vi "SELECT Income and Expenses.vi"(8 "error in (no error)":errorcluster, 9 "Month":T1, 10 "YYYY":i32, 11 "Database in":refnum<class "Database.lvclass">) -> (0 "error out":errorcluster, 1 "Total Expenses":dbl, 2 "Total Income":dbl, 3 "Database out":refnum<class "Database.lvclass">)   [LabVIEW 2018, in "Database.lvclass"]
uses:
  Database.lvclass
  Month.ctl
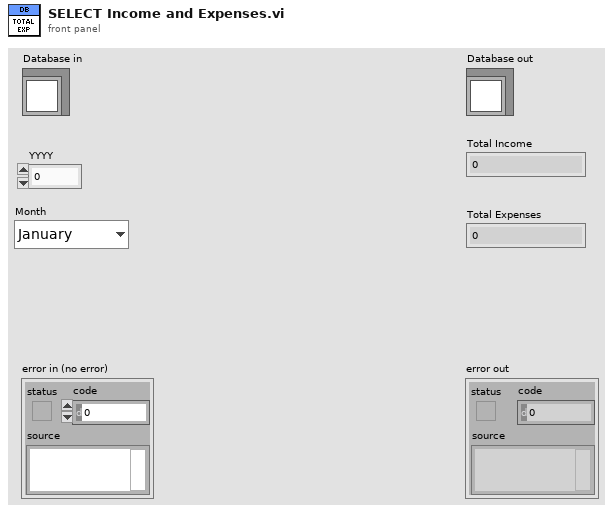
[diagram p1: front panel]
types:
  T1 = typedef "Database.lvclass/Month.ctl" = enum16{"January", "February", "March", "April", "May", "June", "July", "August", "September", "October", "November", "December"}
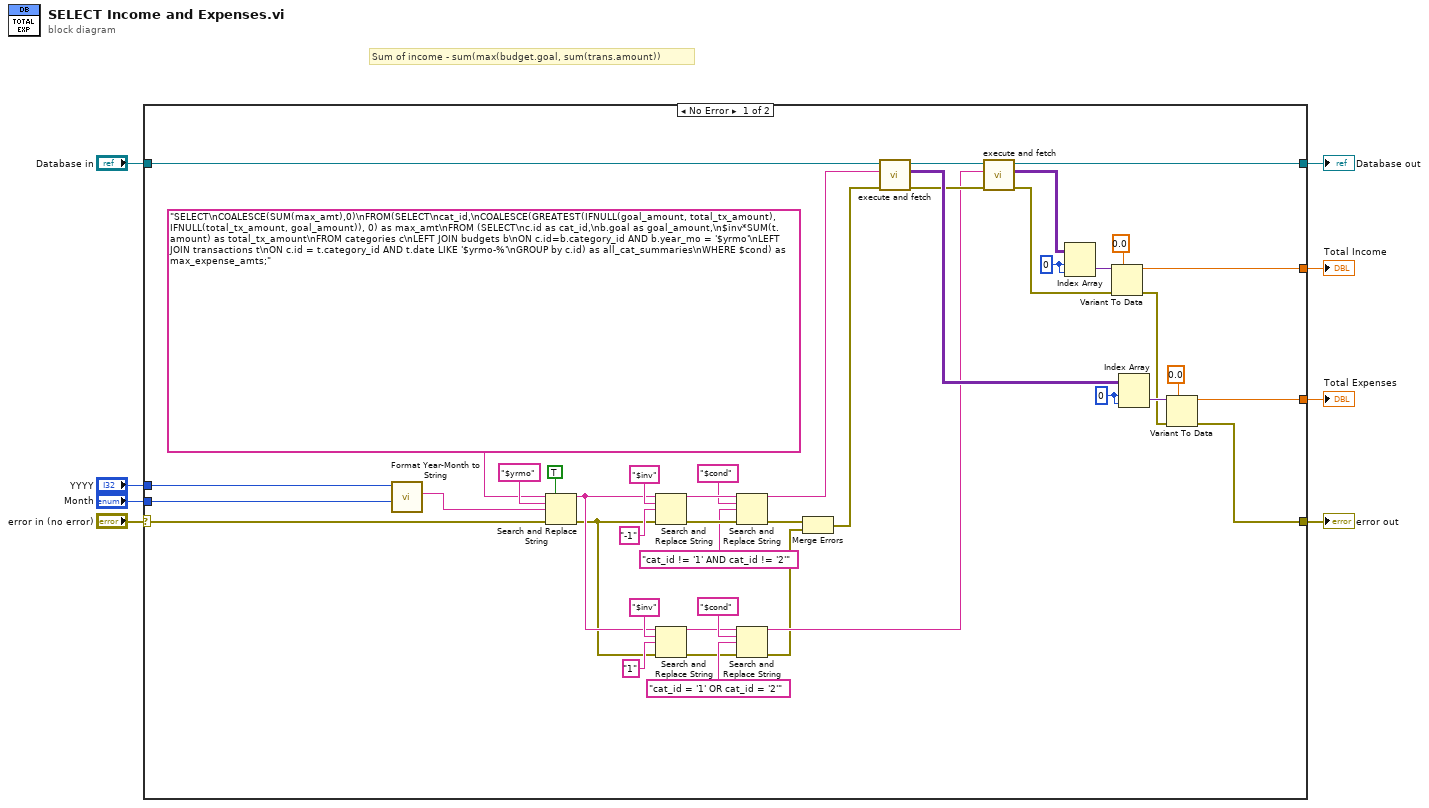
[diagram p0: block diagram]
diagram:
  # "Sum of income - sum(max(budget.goal, sum(trans.amount))"
  n1 = case shown="No Error" "error in (no error)" {
    selector: "error in (no error)" -> [w25 w53]
    tunnel: [w41 w53] -> w7
    tunnel: [w14 w52] -> w5
    tunnel: "Database in" -> [w51 w52]
    tunnel: "YYYY" -> [w50 _]
    tunnel: "Month" -> [w49 _]
    tunnel: [w40 _] -> w2
    tunnel: [w15 _] -> w1
    frame No Error {
      w17 = 0 ("index (row)")
      w44 = 0 ("index (row)")
      n2 = call "Format Year-Month to String.vi"("Month"=w49, "YYYY"=w50) -> ("Year-Mo"=w46:string)  [unwired: 9 in]
      n3 = Search and Replace String(replace all?=TRUE ("replace all? (F)"), input string="SELECT\nCOALESCE(SUM(max_amt),0)\nFROM(SELECT\ncat_id,\nCOALESCE(GREATEST(IFNULL(goal_amount, total_tx_amount), IFNULL(total_tx_amount, goal_amount)), 0) as max_amt\nFROM (SELECT\nc.id as cat_id,\nb.goal as goal_amount,\n$inv*SUM(t.amount) as total_tx_amount\nFROM categories c\nLEFT JOIN budgets b\nON c.id=b.category_id AND b.year_mo = '$yrmo'\nLEFT JOIN transactions t\nON c.id = t.category_id AND t.date LIKE '$yrmo-%'\nGROUP by c.id) as all_cat_summaries\nWHERE $cond) as max_expense_amts;", search string="$yrmo", replace string=w46, error in=w25) -> (result string=w24:string, error out=w23:errorcluster)  [unwired: 3 in, 2 out]
      n4 = Search and Replace String(input string=w24, search string="$inv", replace string="-1" ("replace string (\"\")"), error in=w23) -> (result string=w37:string, error out=w36:errorcluster)  [unwired: 4 in, 2 out]
      n5 = Search and Replace String(input string=w24, search string="$inv", replace string="1" ("replace string (\"\")"), error in=w23) -> (result string=w29:string, error out=w30:errorcluster)  [unwired: 4 in, 2 out]
      n6 = Search and Replace String(input string=w37, search string="$cond", replace string="cat_id != '1' AND cat_id != '2'" ("replace string (\"\")"), error in=w36) -> (result string=w33:string, error out=w11:errorcluster)  [unwired: 4 in, 2 out]
      n7 = Search and Replace String(input string=w29, search string="$cond", replace string="cat_id = '1' OR cat_id = '2'" ("replace string (\"\")"), error in=w30) -> (result string=w20:string, error out=w10:errorcluster)  [unwired: 4 in, 2 out]
      n8 = Merge Errors(w11, w10) -> (w9:errorcluster)
      n9 = call "execute and fetch.vi"("error in (no error)"=w9, "SQL query"=w33, "Database in"=w51) -> ("error out"=w21:errorcluster, "recordset data"=w45:variant[][], "Database out"=w22:refnum<class "Database.lvclass">)  [unwired: 5 in, 1 out]
      n10 = call "execute and fetch.vi"("error in (no error)"=w21, "SQL query"=w20, "Database in"=w22) -> ("error out"=w13:errorcluster, "recordset data"=w16:variant[][], "Database out"=w14:refnum<class "Database.lvclass">)  [unwired: 5 in, 1 out]
      n11 = Index Array(array=w16, index (row)=w17, index (col)=w17) -> (element=w18:variant)
      n12 = Variant To Data(error in=w13, type=0.0, Variant=w18) -> (data=w15:dbl, error out=w12:errorcluster)
      n13 = Index Array(array=w45, index (row)=w44, index (col)=w44) -> (element=w43:variant)
      n14 = Variant To Data(error in=w12, type=0.0, Variant=w43) -> (data=w40:dbl, error out=w41:errorcluster)
    }
    frame Error {
    }
  }
  "error out" <- w7
  "Database out" <- w5
  "Total Expenses" <- w2
  "Total Income" <- w1
